vi "Actor Core.vi"(8 "error in":errorcluster, 11 "Nested in":refnum<class "[V] Sys Cfg Base.lvclass">) -> (0 "error out":errorcluster, 3 "Actor out":refnum<class "Actor.lvclass">)   [LabVIEW 2020, in "[V] Sys Cfg Base.lvlib" / "[V] Sys Cfg Base.lvclass"]
doc: "(<B>Filename</B>: Actor Framework.lvlib:Actor.lvclass:Actor Core.vi)\n\nReceives messages to the actor, reacts to them, and initiates any error handling that may shut the actor down.\n\nDescendant classes may override this VI to append parallel tasks for the actor to complete while it handles messages. Overrides use the Call Parent Method node."
uses:
  [V] Sys Cfg Base.lvclass
  <vilib>/ActorFramework/Actor/Actor.lvclass
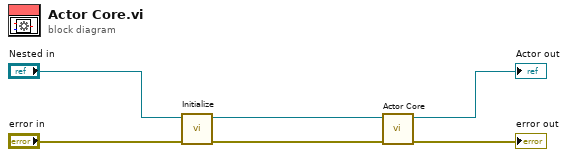
[diagram p0: block diagram]
diagram:
  n1 = call "Initialize.vi"("error in (no error)"="error in", "[V] Sys Cfg Base in"="Nested in") -> ("error out"=w1:errorcluster, "[V] Sys Cfg Base out"=w2:refnum<class "[V] Sys Cfg Base.lvclass">)  [unwired: 8 in]
  n2 = call-parent "Actor Core.vi"("error in"=w1, "Actor in"=w2) -> ("error out"=→"error out":errorcluster, "Actor out"=→"Actor out":refnum<class "Actor.lvclass">)  [unwired: 8 in]
